vi "Aquisition Loop.vi"(8 "error out":errorcluster, 9 "notifier out":refnum<notifier>, 11 "queue out":refnum<queue>) -> ()   [LabVIEW 2015]
uses:
  Finite Acquisition - Solution/TypeDefs/Queue Data.ctl
  Finite Acquisition - Solution/SubVIs/App Data.vi
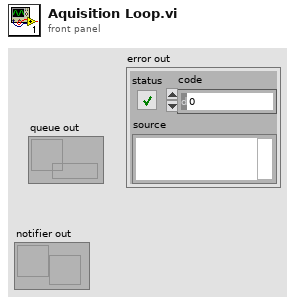
[diagram p1: front panel]
types:
  T1 = typedef "Queue Data.ctl" = cluster{"Action":string}
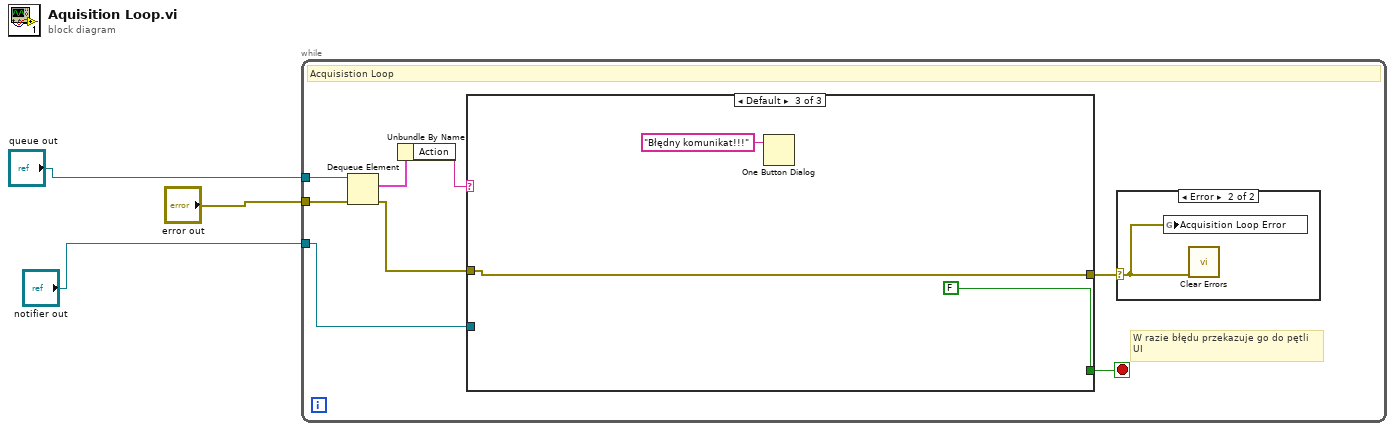
[diagram p0: block diagram]
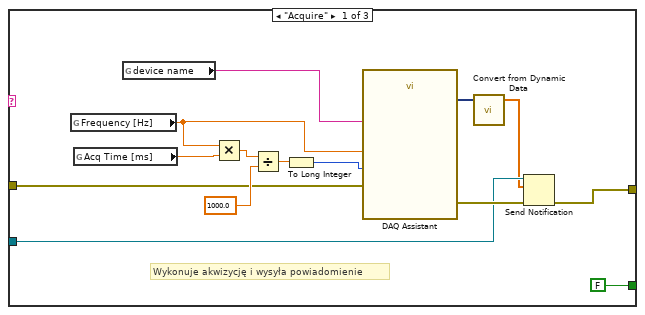
[diagram p3: hidden frame]
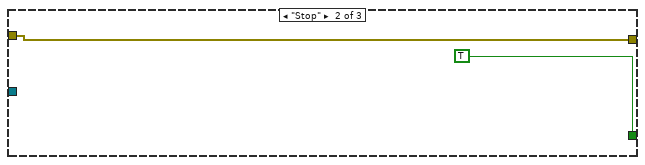
[diagram p4: hidden frame]
diagram:
  n1 = while {
    tunnel: "error out" -> [w9]
    tunnel: "queue out" -> [w8]
    tunnel: "notifier out" -> [w4]
    stop <- w6 stop-if-true
    # "W razie błędu przekazuje go do pętli\nUI"
    # "Acquisistion Loop"
    n2 = Dequeue Element(queue=w8, error in (no error)=w9) -> (element=w11:T1, error out=w7:errorcluster)  [unwired: 1 in, 2 out]
    n3 = Unbundle By Name(w11) -> ("Action"=w10:string)
    n4 = case shown="Default" w10 {
      tunnel: w7 -> [w20 w27 w30]
      tunnel: [FALSE TRUE FALSE] -> w6
      tunnel: [w16 w27 w30] -> w5
      tunnel: w4 -> [w15 _ _]
      frame "Acquire" {
        # "Wykonuje akwizycję i wysyła powiadomienie"
        n5 = global read "App Data.vi" "Frequency [Hz]"() -> (w26:dbl)
        n6 = global read "App Data.vi" "Acq Time [ms]"() -> (w25:dbl)
        n7 = global read "App Data.vi" "device name"() -> (w18:tag)
        n8 = Multiply(x=w26, y=w25) -> (x*y=w24:dbl)
        n9 = Divide(x=w24, y=1000.0) -> (x/y=w22:dbl)
        n10 = To Long Integer(number=w22) -> (32bit integer=w21:i32)
        n11 = call "DAQ Assistant"("rate"=w26, "number of samples"=w21, "error in"=w20, "device name"=w18) -> ("data"=w14:dynamicdata, "error out"=w17:errorcluster)  [unwired: 13 in, 1 out]
        n12 = call "Convert from Dynamic Data"("Dynamic Data Type"=w14) -> ("Array"=w13:dbl[])  [unwired: 3 in]
        n13 = Send Notification(notification=w13, notifier=w15, error in (no error)=w17) -> (error out=w16:errorcluster)  [unwired: 1 out]
      }
      frame "Stop" {
      }
      frame Default {
        n14 = One Button Dialog(message="Błędny komunikat!!!") -> ()  [unwired: 1 in, 1 out]
      }
    }
    n15 = case shown="Error" w5 {
      selector: w5 -> [_ w12]
      frame No Error {
      }
      frame Error {
        n16 = global write "App Data.vi" "Acquisition Loop Error"(w12) -> ()
        n17 = call <vilib>:"Clear Errors.vi"("error in (no error)"=w12) -> ()  [unwired: 5 in, 2 out]
      }
    }
  }
